vi "Read Event.vi"(8 "error in (no error)":errorcluster, 11 "EventLogHandle in":refnum<class "EventLogHandle.lvclass">) -> (0 "error out":errorcluster, 2 "Event":refnum<user-event>, 3 "EventLogHandle out":refnum<class "EventLogHandle.lvclass">)   [LabVIEW 2024, in "EventLogHandle.lvclass"]
uses:
  EventLogHandle.lvclass
  Record/LogRecord.lvclass
  EventLogHandle.lvclass/EventLogHandle.ctl
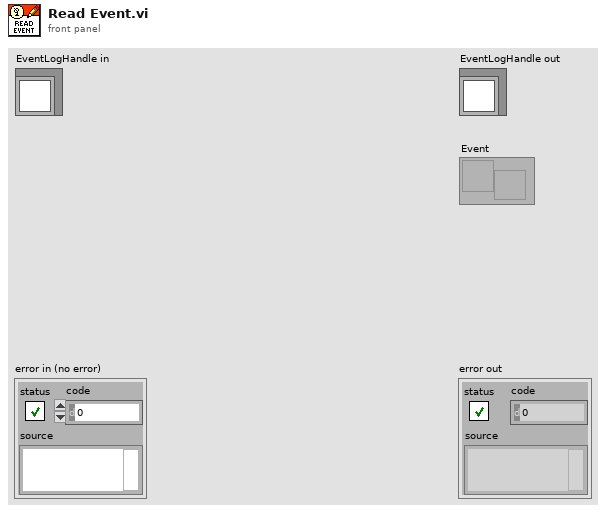
[diagram p1: front panel]
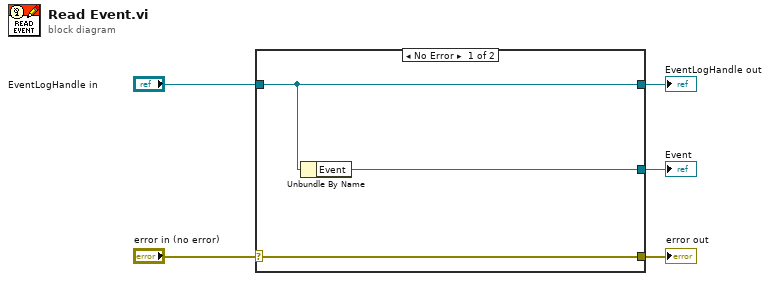
[diagram p0: block diagram]
diagram:
  n1 = case shown="No Error" "error in (no error)" {
    selector: "error in (no error)" -> [w8 w9]
    tunnel: [w8 w9] -> w4
    tunnel: [w7 w10] -> w2
    tunnel: "EventLogHandle in" -> [w7 w10]
    tunnel: [w6 _] -> w1
    frame No Error {
      n2 = Unbundle By Name(w7) -> ("Event"=w6:refnum<user-event>)
    }
    frame Error {
    }
  }
  "error out" <- w4
  "EventLogHandle out" <- w2
  "Event" <- w1
